vi "DoubleSolenoidPulse_Example.vi"() -> ()   [LabVIEW 2019]
uses:
  <vilib>/Rock Robotics/WPI/ThirdParty/JAS_Junk/TrajLib/VI/Util_GetTime_U32.vi
  <vilib>/Rock Robotics/WPI/ThirdParty/JAS_Junk/TrajLib/Timer_New.vi
  <vilib>/Rock Robotics/WPI/ThirdParty/JAS_Junk/TrajLib/VI/TimeInterpBoolean_New.vi
  <vilib>/Rock Robotics/WPI/ThirdParty/JAS_Junk/TrajLib/VI/TimeInterpBoolean_AddSample.vi
  <vilib>/Rock Robotics/WPI/ThirdParty/JAS_Junk/TrajLib/VI/TimeInterpBoolean_GetSample.vi
  <vilib>/Rock Robotics/WPI/ThirdParty/JAS_Junk/TrajLib/VI/TimeInterpBoolean_SetMaxTime.vi
  <vilib>/Rock Robotics/WPI/ThirdParty/JAS_Junk/TrajLib/VI/TimeInterpBoolean_CleanUp.vi
  <vilib>/Rock Robotics/WPI/ThirdParty/JAS_Junk/TrajLib/VI/Util_GetTime_U64.vi
  <vilib>/Utility/semaphor.llb/Obtain Semaphore Reference.vi
  <vilib>/Rock Robotics/WPI/ThirdParty/JAS_Junk/TrajLib/Timer_Reset.vi
  <vilib>/Rock Robotics/WPI/ThirdParty/JAS_Junk/TrajLib/Timer_Start.vi
  <vilib>/Rock Robotics/WPI/ThirdParty/JAS_Junk/TrajLib/Timer_HasPeriodPassedOnce.vi
  <vilib>/gmath/interp.llb/Search Ordered Table.vi
  <vilib>/Rock Robotics/WPI/ThirdParty/JAS_Junk/TrajLib/Trajectory_Library.lvlib
panel:
  out "Quad Encoder Direction":string
  out "Waveform Chart":cluster{i16, i16}(graph)
  out "IsPresent":bool
  out "Delayed Output":bool
  out "Output":bool
  in  "Period (ms)":dbl=1800.0
  in  "Delay (ms)":dbl=600.0
  # "DIGITAL DELAY EXAMPLE"
  # "Set at 1/3 of period for fwd, 2/3 of period for reverse."
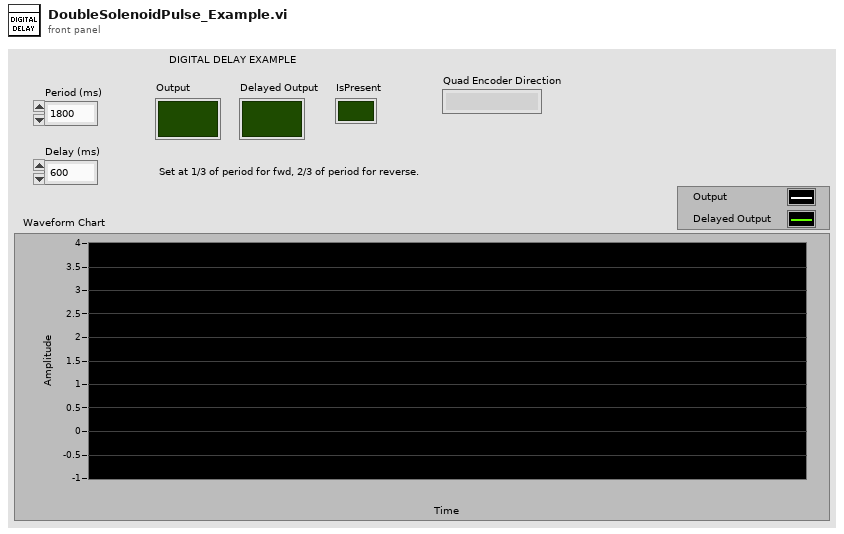
[diagram p1: front panel]
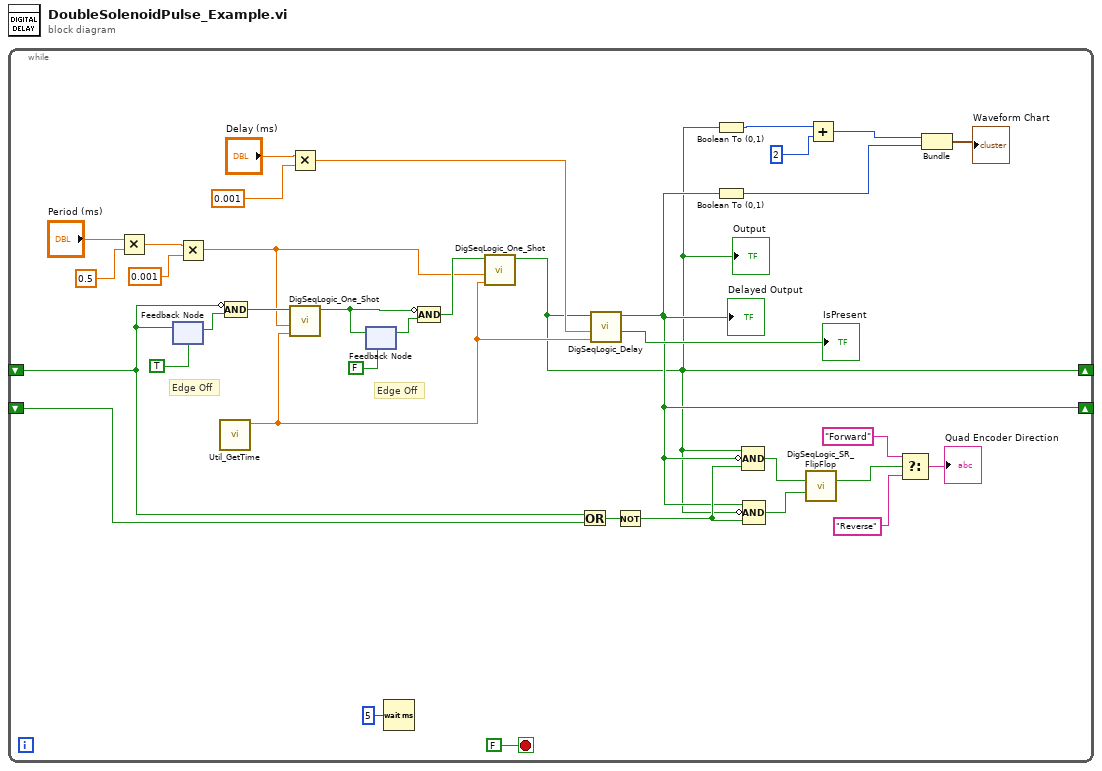
[diagram p0: block diagram]
diagram:
  n1 = while {
    shift-right: [w4] -> _
    shift-left: _ -> [w11]
    shift-right: [w5] -> _
    shift-left: _ -> [w10]
    stop <- FALSE stop-if-true
    # "Edge Off"
    # "Edge Off"
    n2 = Multiply(x="Period (ms)", y=0.5) -> (x*y=w32:dbl)
    n3 = feedback-in #1(w11) -> ()
    n4 = feedback #1(TRUE ("Output")) -> (w29:bool)
    n5 = Multiply(x=w32, y=0.001) -> (x*y=w23:dbl)
    n6 = call <vilib>:"Util_GetTime.vi"() -> ("FPGA_Time_Seconds"=w22:dbl)  [unwired: 9 in, 2 out]
    n7 = Compound Arithmetic op=AND(invert w11, w29) -> (w28:bool)
    n8 = Multiply(x="Delay (ms)", y=0.001) -> (x*y=w19:dbl)
    n9 = call <vilib>:"DigSeqLogic_One_Shot.vi"("Time"=w22, "OneShot"=w23, "Input"=w28) -> ("Output"=w27:bool)  [unwired: 7 in, 1 out]
    n10 = feedback #2(FALSE ("Output")) -> (w26:bool)
    n11 = feedback-in #2(w27) -> ()
    n12 = Wait (ms)(milliseconds to wait=u32 5) -> ()  [unwired: 1 out]
    n13 = Compound Arithmetic op=AND(invert w27, w26) -> (w24:bool)
    n14 = call <vilib>:"DigSeqLogic_One_Shot.vi"("Time"=w22, "OneShot"=w23, "Input"=w24) -> ("Output"=w4:bool)  [unwired: 7 in, 1 out]
    "Output" <- w4
    n15 = Or(x=w11, y=w10) -> (x .or. y?=w12:bool)
    n16 = call <vilib>:"DigSeqLogic_Delay.vi"("Time"=w22, "Delay Time"=w19, "Input"=w4) -> ("IsPresent"=→"IsPresent":bool, "Output"=w5:bool)  [unwired: 7 in]
    "Delayed Output" <- w5
    n17 = Not(x=w12) -> (.not. x?=w6:bool)
    n18 = Boolean To (0,1)(Boolean=w4) -> (0, 1=w15:i16)
    n19 = Boolean To (0,1)(Boolean=w5) -> (0, 1=w13:i16)
    n20 = Compound Arithmetic op=AND(w4, invert w5, w6) -> (w3:bool)
    n21 = Compound Arithmetic op=AND(w5, invert w4, w6) -> (w2:bool)
    n22 = call <vilib>:"DigSeqLogic_SR_FlipFlop.vi"("Set"=w3, "Reset"=w2) -> ("Output"=w9:bool)  [unwired: 12 in, 1 out]
    n23 = Add(x=w15, y=i16 2) -> (x+y=w14:i16)
    n24 = Select(t="Forward", s=w9, f="Reverse") -> (s? t:f=→"Quad Encoder Direction":string)
    n25 = Bundle(w14, w13) -> (→"Waveform Chart":cluster{i16, i16})  [unwired: 1 in]
  }
